vi "Formal Check Rows by Int.vi"(10 "Sudoku Formal In":T1, 11 "Sudoku Int":u8[][](array[numeric])) -> (2 "Sudoku Formal Out":T1, 3 "Is Modify":bool)   [LabVIEW 2015, in "Sudoku Library.lvlib"]
doc: "Created IvanLis by LabVIEW Portal\nProfile: http://labviewportal.org/memberlist.php?mode=viewprofile&u=987\neMail: IvanLisanov@gMail.com\nTelegram: https://t.me/IvanLis"
uses:
  Sudoku Library.lvlib
  TypeDef/Sudoku Formal.ctl
  TypeDef/Cell Formal.ctl
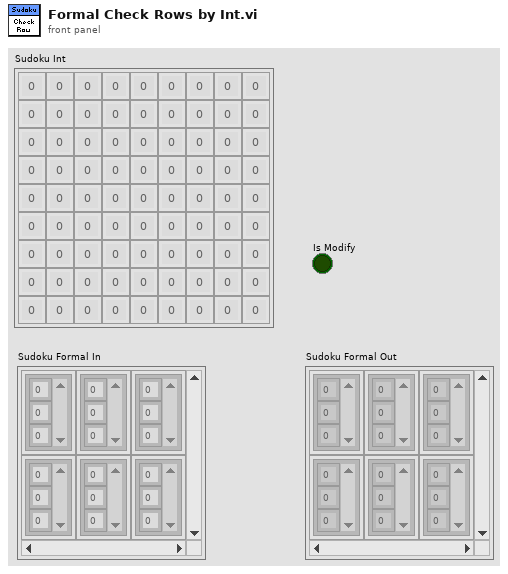
[diagram p1: front panel]
types:
  T1 = typedef "Sudoku Library.lvlib/Sudoku Formal.ctl" = T2[][]
  T2 = typedef "Sudoku Library.lvlib/Cell Formal.ctl" = cluster{"Variant":u8[]}
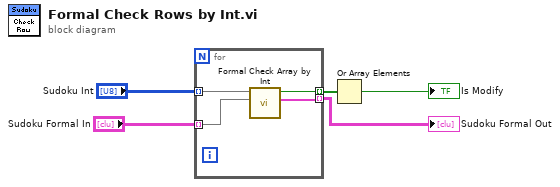
[diagram p0: block diagram]
diagram:
  n1 = for {
    tunnel: "Sudoku Int" -> [w9] mode=indexing
    tunnel: "Sudoku Formal In" -> [w8] mode=indexing
    tunnel: [w7] -> w5 mode=indexing
    tunnel: [w6] -> w1 mode=indexing
    n2 = call "Formal Check Array by Int.vi"("Array Formal In"=w8, "Array In"=w9) -> ("Array Formal Out"=w6:T2[], "Is Modify"=w7:bool)  [unwired: 8 in]
  }
  "Sudoku Formal Out" <- w1
  n3 = Or Array Elements(Boolean array=w5) -> (logical OR=→"Is Modify":bool)
